vi "Draw.vi"(8 "Error In":errorcluster, 11 "Pixel In":refnum<class "String.lvclass">) -> (0 "Error Out":errorcluster, 2 "Element To Display":T1[](array[typedef]), 3 "Pixel Out":refnum<class "String.lvclass">)   [LabVIEW 2019, in "String.lvclass"]
uses:
  String.lvclass
  C:/Users/goo13/Documents/GIT Local/myRIO-Neopixel/Source/RT/Display Element/Display Element.lvclass
  Display Element/Public/Controls/Pixel.ctl
  Display Element/Public/Controls/Vector.ctl
  Display Element/Display Element.lvclass
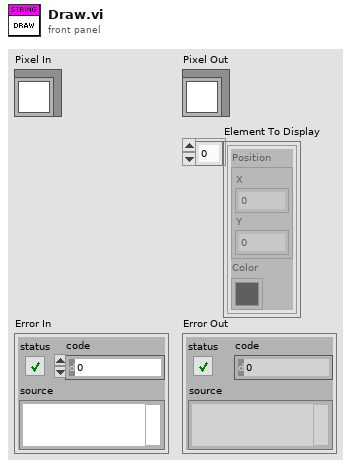
[diagram p1: front panel]
types:
  T1 = typedef "Display Element.lvclass/Pixel.ctl" = cluster{"Position":T2, "Color":u32}
  T2 = typedef "Display Element.lvclass/Vector.ctl" = cluster{"X":i32, "Y":i32}
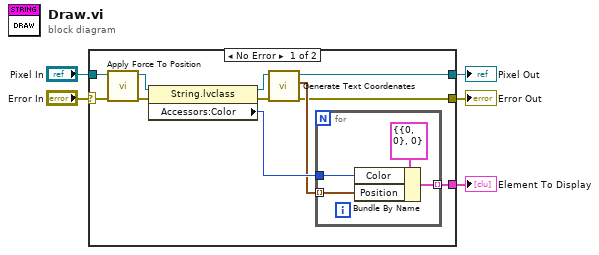
[diagram p0: block diagram]
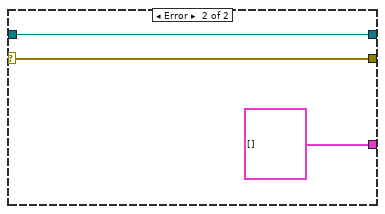
[diagram p2: hidden frame]
diagram:
  n1 = case shown="No Error" "Error In" {
    selector: "Error In" -> [w13 w23]
    tunnel: "Pixel In" -> [w14 w22]
    tunnel: [w6 w23] -> w3
    tunnel: [w8 w22] -> w2
    tunnel: [w15 T1[] []] -> w1
    frame No Error {
      n2 = call-dynamic "Apply Force To Position.vi"("Error In"=w13, "Display Element In"=w14) -> ("Error Out"=w11:errorcluster, "Display Element Out"=w12:refnum<class "String.lvclass">)  [unwired: 8 in]
      n3 = property class="String.lvclass"(reference=w12, error in=w11) -> (reference out=w10:refnum<class "String.lvclass">, error out=w9:errorcluster, "Accessors:Color"=w16:u32)
      n4 = call "Generate Text Coordenates.vi"("Error In"=w9, "Pixel In"=w10) -> ("Error Out"=w6:errorcluster, "Element To Display"=w7:T2[], "Pixel Out"=w8:refnum<class "String.lvclass">)  [unwired: 7 in]
      n5 = for {
        tunnel: w7 -> [w19] mode=indexing
        tunnel: w16 -> [w17]
        tunnel: [w18] -> w15 mode=indexing
        n6 = Bundle By Name(cluster=T1 {"Position"={"X"=0, "Y"=0}, "Color"=0} ("Pixel"), "Color"=w17, "Position"=w19) -> (w18:T1)
      }
    }
    frame Error {
    }
  }
  "Pixel Out" <- w2
  "Error Out" <- w3
  "Element To Display" <- w1
